vi "ACT_limit_setpoint_and_control.vi"(0 "MD420.lvclass in":refnum<class "MD420.lvclass">, 1 "ACT upper limit":dbl, 2 "ACT Setpoint":dbl, 3 "Apply ACT SP":bool, 4 "Block D withd":bool, 5 "All D in L":bool, 6 "Increase ACT limit Setpoint":bool, 7 "error out":errorcluster) -> (20 "MD420.lvclass out":refnum<class "MD420.lvclass">, 22 "Release +0,6 K/min":bool, 23 "ACT limit Setpoint":dbl, 24 "ACT limit Setpoint\ndecreased":bool, 27 "error out":errorcluster)   [LabVIEW 2022 SP3, in "MD420.lvclass"]
uses:
  MD420.lvclass
  MD420.lvclass/MD420.ctl
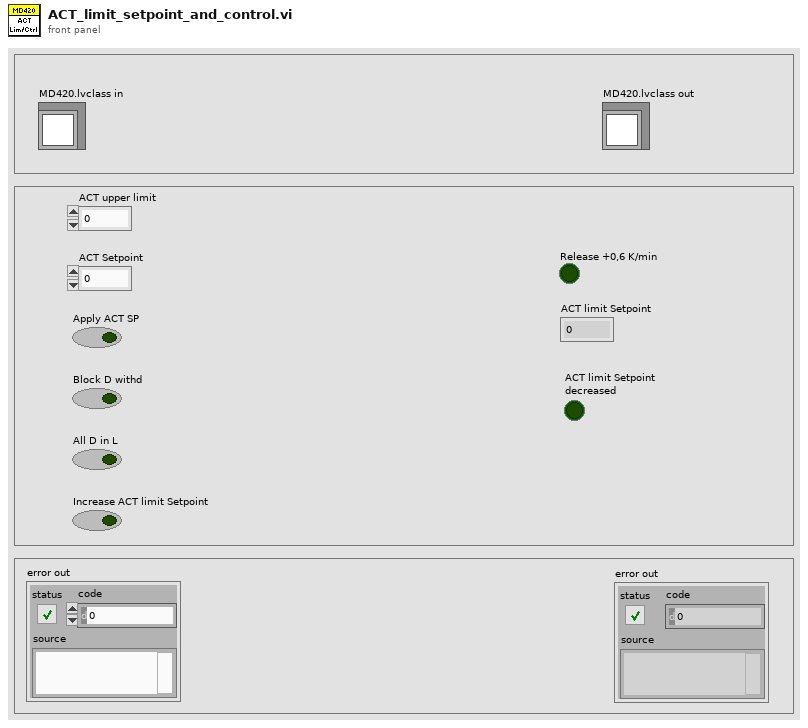
[diagram p1: front panel]
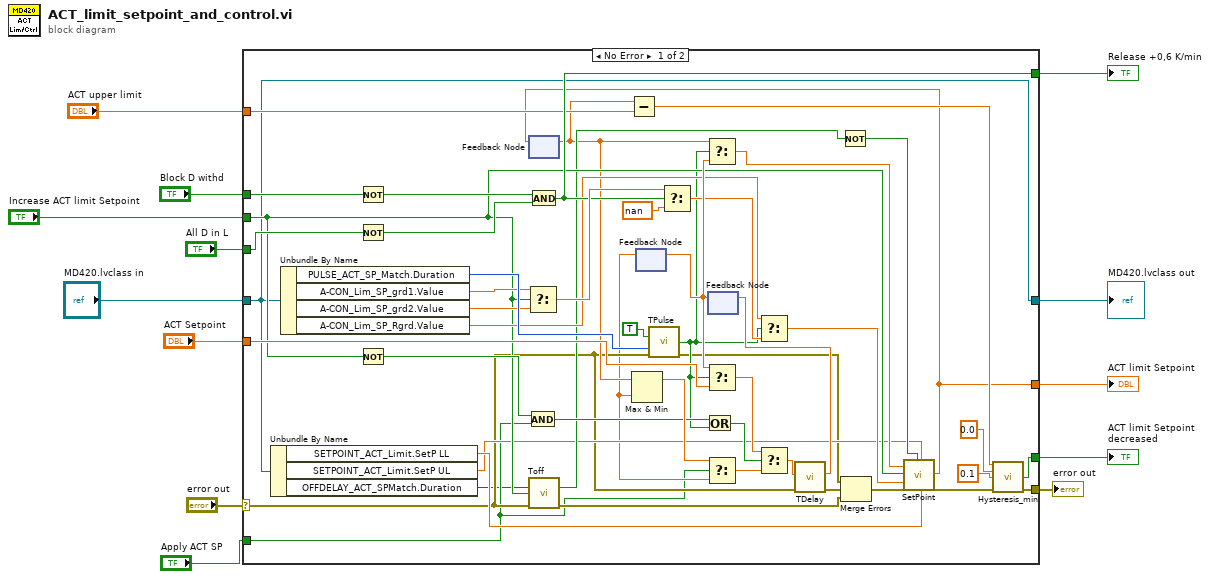
[diagram p0: block diagram]
diagram:
  n1 = case shown="No Error" "error out" {
    selector: "error out" -> [w24 w64]
    tunnel: [w18 w64] -> w12
    tunnel: "ACT Setpoint" -> [w62 _]
    tunnel: "Apply ACT SP" -> [w16 _]
    tunnel: "Block D withd" -> [w46 _]
    tunnel: "All D in L" -> [w45 _]
    tunnel: "Increase ACT limit Setpoint" -> [w39 _]
    tunnel: "MD420.lvclass in" -> [w14 w63]
    tunnel: [w42 _] -> w5
    tunnel: "ACT upper limit" -> [w31 _]
    tunnel: [w28 _] -> w3
    tunnel: [w27 _] -> w2
    tunnel: [w14 w63] -> w1
    frame No Error {
      n2 = Unbundle By Name(w14) -> ("SETPOINT_ACT_Limit.SetP LL"=w34:dbl, "SETPOINT_ACT_Limit.SetP UL"=w33:dbl, "OFFDELAY_ACT_SPMatch.Duration"=w15:i32)
      n3 = Unbundle By Name(w14) -> ("PULSE_ACT_SP_Match.Duration"=w57:i32, "A-CON_Lim_SP_grd1.Value"=w50:dbl, "A-CON_Lim_SP_grd2.Value"=w49:dbl, "A-CON_Lim_SP_Rgrd.Value"=w41:dbl)
      n4 = Not(x=w46) -> (.not. x?=w47:bool)
      n5 = Not(x=w45) -> (.not. x?=w48:bool)
      n6 = Not(x=w39) -> (.not. x?=w55:bool)
      n7 = Select(t=w50, s=w39, f=w49) -> (s? t:f=w44:dbl)
      n8 = And(x=w55, y=w16) -> (x .and. y?=w54:bool)
      n9 = feedback #1() -> (w29:dbl)  [unwired: 1 in]
      n10 = And(x=w47, y=w48) -> (x .and. y?=w42:bool)
      n11 = call "Toff.vi"("preset time (ms)"=w15, "input"=w39, "error in"=w24) -> ("off"=w36:bool, "error out"=w21:errorcluster)  [unwired: 10 in, 1 out]
      n12 = Subtract(x=w29, y=w31) -> (x-y=w32:dbl)
      n13 = feedback #2() -> (w17:dbl)  [unwired: 1 in]
      n14 = Max & Min(x=w29, y=w17) -> (max(x,y)=w61:dbl)  [unwired: 1 out]
      n15 = call "TPulse.vi"("trigger"=TRUE ("input"), "TPulse"=w57, "error in"=w24) -> ("output"=w30:bool, "error out"=w23:errorcluster)  [unwired: 10 in, 1 out]
      n16 = Select(t=w44, s=w42, f=nan) -> (s? t:f=w40:dbl)
      n17 = Or(x=w54, y=w30) -> (x .or. y?=w53:bool)
      n18 = Select(t=w61, s=w16, f=w17) -> (s? t:f=w60:dbl)
      n19 = feedback #3() -> (w51:dbl)  [unwired: 1 in]
      n20 = feedback-in #2(w51) -> ()
      n21 = Select(t=w29, s=w30, f=w51) -> (s? t:f=w38:dbl)
      n22 = Select(t=w51, s=w30, f=w62) -> (s? t:f=w59:dbl)
      n23 = Select(t=w41, s=w30, f=w40) -> (s? t:f=w35:dbl)
      n24 = Select(t=w59, s=w53, f=w60) -> (s? t:f=w56:dbl)
      n25 = call "TDelay.vi"("Error in"=w24, "input"=w56) -> ("Error out"=w22:errorcluster, "output"=w52:dbl)  [unwired: 8 in]
      n26 = feedback-in #3(w52) -> ()
      n27 = Not(x=w36) -> (.not. x?=w37:bool)
      n28 = Merge Errors(w23, w22, w21) -> (w20:errorcluster)
      n29 = call "SetPoint.vi"("IAd(AI2)"=w38, "I+(BI2)"=w39, "Igrd(AI1)"=w35, "error in"=w20, "IC(BI3)"=w37, "SetP UL"=w33, "SetP LL"=w34) -> ("Output (AO1)"=w28:dbl, "error out"=w19:errorcluster)  [unwired: 19 in]
      n30 = feedback-in #1(w28) -> ()
      n31 = call "Hysteresis_min.vi"("input"=w32, "Min"=0.0, "H"=0.1, "error in"=w19) -> ("Deviation"=w27:bool, "error out"=w18:errorcluster)  [unwired: 10 in]
    }
    frame Error {
    }
  }
  "error out" <- w12
  "Release +0,6 K/min" <- w5
  "ACT limit Setpoint" <- w3
  "ACT limit Setpoint\ndecreased" <- w2
  "MD420.lvclass out" <- w1
